vi "Amount Editor GUI.vi"(8 "error in (no error)":errorcluster, 11 "Input Amount":dbl) -> (0 "error out":errorcluster, 2 "UserConfirm?":bool, 3 "Output Amount":dbl)   [LabVIEW 2018]
panel:
  in  "Ok":bool
  in  "Amount":dbl
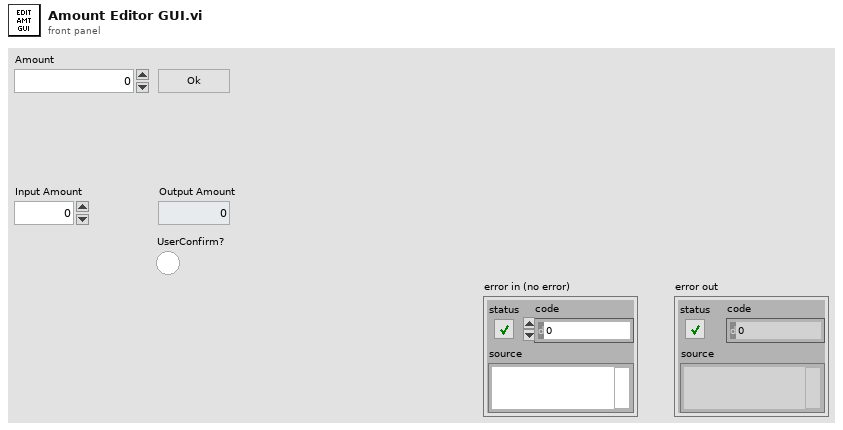
[diagram p1: front panel]
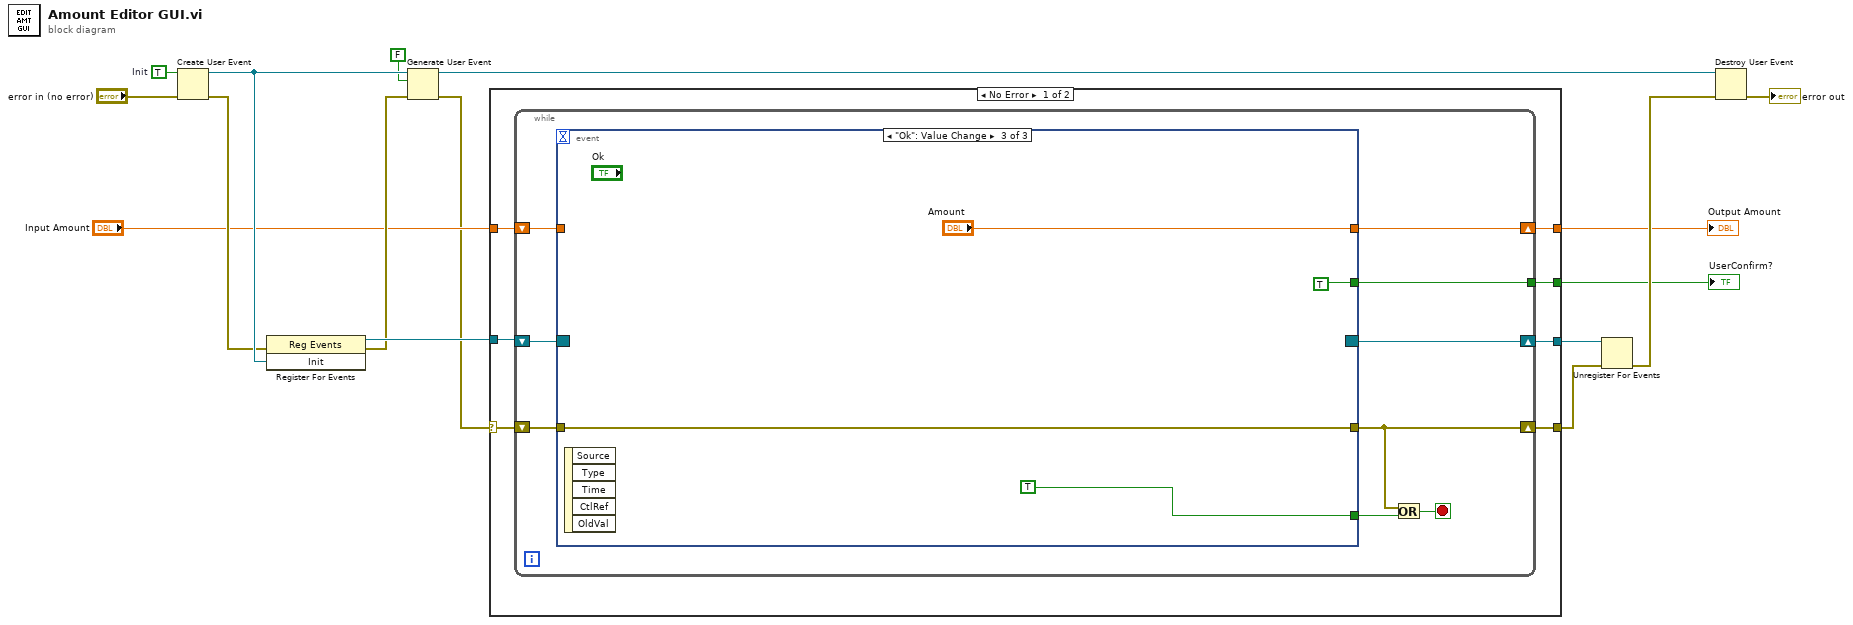
[diagram p0: block diagram]
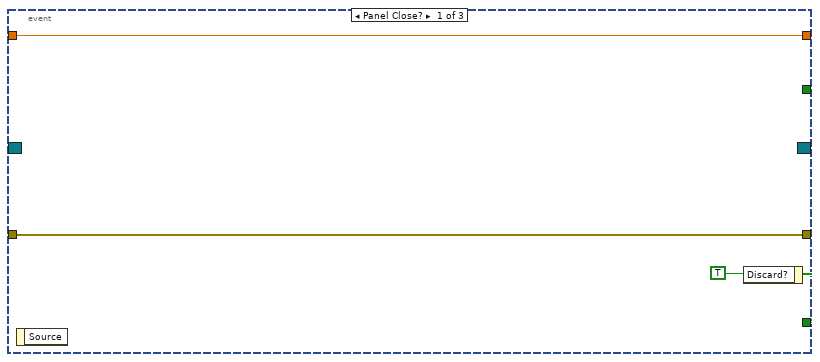
[diagram p2: hidden frame]
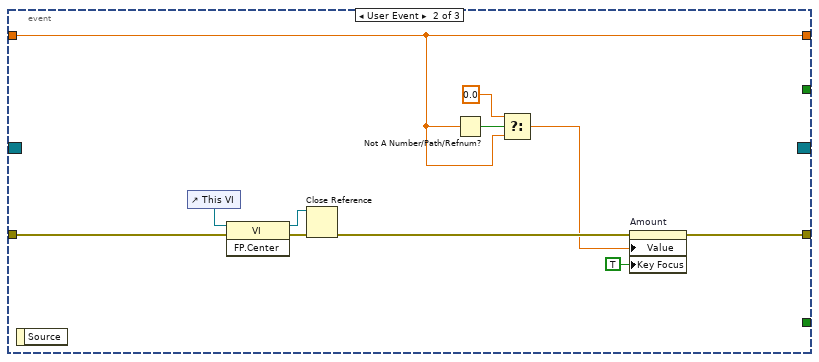
[diagram p3: hidden frame]
diagram:
  w16 = TRUE  # Init
  n1 = Create User Event(user event datatype=w16, error in="error in (no error)") -> (user event=w14:refnum<user-event>, error out=w11:errorcluster)
  n2 = register-events(error in=w11, w14) -> (reference out=w15:refnum<event-registration>, error out=w13:errorcluster)  [unwired: 1 in]
  n3 = Generate User Event(user event=w14, event data cluster=FALSE ("event data"), error in=w13) -> (user event out=w10:refnum<user-event>, error out=w1:errorcluster)  [unwired: 1 in]
  n4 = case shown="No Error" w1 {
    selector: w1 -> [w17 w53]
    tunnel: w15 -> [w23 w52]
    tunnel: [w22 w52] -> w9
    tunnel: [w21 w53] -> w8
    tunnel: [w20 w51] -> w4
    tunnel: "Input Amount" -> [w19 w51]
    tunnel: [w18 _] -> w2
    frame No Error {
      n5 = while {
        shift-right: [w30] -> w22
        shift-left: w23 -> [w32]
        shift-right: [w29] -> w21
        shift-left: w17 -> [w31]
        tunnel: [w24] -> w18
        shift-right: [w26] -> w20
        shift-left: w19 -> [w25]
        stop <- w27 stop-if-true
        n6 = event shown="[2] \"Ok\": Value Change" {
          selector: w32 -> [_ _ _]
          dyn-events: [_ _ _] -> w30
          timeout: _ -> [_ _ _]
          tunnel: [w35 _ TRUE ("Discard?")] -> w28
          tunnel: w31 -> [w34 w45 w49]
          tunnel: [w34 w42 w49] -> w29
          tunnel: [w33 w38 "Amount"] -> w26
          tunnel: w25 -> [w33 w38 _]
          tunnel: [_ _ TRUE ("Discard?")] -> w24
          event Panel Close? {
            w35 = TRUE ("Discard?")
            n7 = event-data() -> ()  [unwired: 1 in, 1 out]
            n8 = event-data("Discard?"=w35) -> ()  [unwired: 1 in, 1 out]
          }
          event User Event {
            n9 = event-data() -> ()  [unwired: 1 in, 1 out]
            n10 = control-ref of="This VI"() -> (w46:refnum<vi>)
            n11 = invoke class="VI" method="FP.Center"(reference=w46, error in=w45) -> (reference out=w43:refnum<vi>, error out=w44:errorcluster)  [unwired: 1 in, 1 out]
            n12 = Close Reference(reference=w43, error in (no error)=w44) -> (error out=w40:errorcluster)
            n13 = Not A Number/Path/Refnum?(number/path/refnum=w38) -> (NaN/Path/Refnum?=w39:bool)
            n14 = Select(t=0.0, s=w39, f=w38) -> (s? t:f=w37:dbl)
            n15 = property on="Amount" class="DigNum (strict)"(error in=w40, "Value"=w37, "Key Focus"=TRUE) -> (error out=w42:errorcluster)  [unwired: 1 in, 1 out]
          }
          event "Ok": Value Change {
            n16 = event-data() -> ()  [unwired: 1 in, 5 out]
          }
        }
        n17 = Or(x=w29, y=w28) -> (x .or. y?=w27:bool)
      }
    }
    frame Error {
    }
  }
  "Output Amount" <- w4
  "UserConfirm?" <- w2
  n18 = Unregister For Events(event registration refnum=w9, error in=w8) -> (error out=w6:errorcluster)
  n19 = Destroy User Event(user event=w10, error in=w6) -> (error out=→"error out":errorcluster)
